vi "Create.vi"(8 "error in (no error)":errorcluster, 9 "multicast_ip":string="224.1.1.1", 10 "buffer":i32=10000, 11 "port":u16) -> (0 "error out":errorcluster, 3 "BME280 out":refnum<class "BME280.lvclass">)   [LabVIEW 2020, in "BME280.lvclass"]
uses:
  BME280.lvclass
  Weather.ctl
  BME280.lvclass/BME280.ctl
  <vilib>/Utility/tcp.llb/UDP Multicast Read-Only Open.vi
  __main.vi
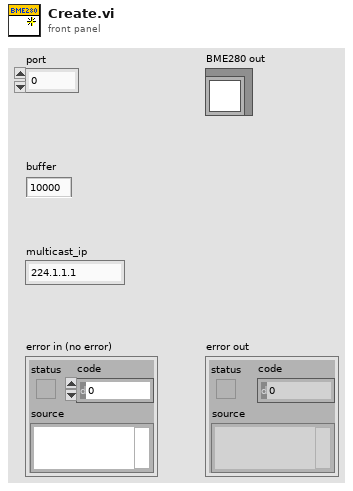
[diagram p1: front panel]
types:
  T1 = typedef "BME280.lvclass/Weather.ctl" = cluster{"temperature":dbl[], "humidity":dbl[], "pressure":dbl[]}
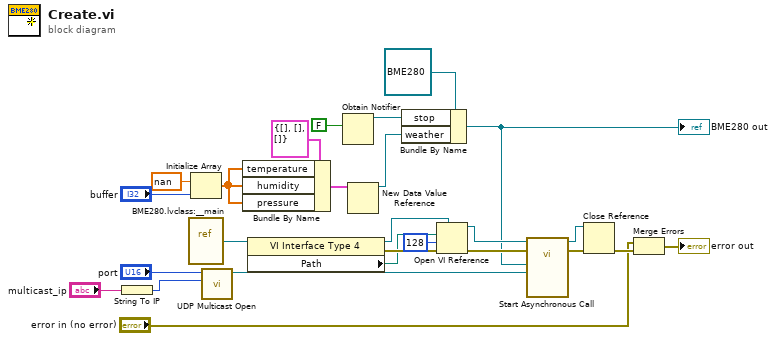
[diagram p0: block diagram]
diagram:
  n1 = String To IP(1:"multicast_ip") -> (0:w1:u32)
  n2 = vi-ref "BME280.lvclass:__main.vi"() -> (w17:refnum<vi>)
  n3 = Initialize Array(nan ("element"), "buffer") -> (w22:dbl[])
  n4 = call-poly <vilib>:"UDP Multicast Open.vi"("multicast addr"=w1, "port"="port") -> ("connection ID"=w2:refnum<k16>)  [unwired: 7 in, 2 out]
  n5 = Bundle By Name(cluster=T1 {"temperature"=[], "humidity"=[], "pressure"=[]} ("weather"), "temperature"=w22, "humidity"=w22, "pressure"=w22) -> (w21:T1)
  n6 = property class="VI Interface Type 4"(reference=w17) -> (reference out=w13:refnum<vi>, error out=w16:errorcluster, "Path"=w15:path)  [unwired: 1 in]
  n7 = Obtain Notifier(notification data type=FALSE) -> (notifier out=w18:refnum<notifier>)  [unwired: 3 in, 2 out]
  n8 = New Data Value Reference(data value=w21) -> (data value reference=w19:refnum<data-value>)  [unwired: 1 in, 1 out]
  n9 = Bundle By Name(cluster=refnum<class "BME280.lvclass"> refnum ("BME280.lvclass"), "stop"=w18, "weather"=w19) -> (w5:refnum<class "BME280.lvclass">)
  "BME280 out" <- w5
  n10 = Open VI Reference(type specifier VI Refnum (for type only)=w13, vi path=w15, options=128, error in (no error)=w16) -> (vi reference=w11:refnum<vi>, error out=w12:errorcluster)  [unwired: 2 in]
  n11 = call-by-ref "Start Asynchronous Call"(reference=w11, error in=w12, "udpCxcn"=w2, "BME280 in"=w5) -> (reference out=w9:refnum<vi>, error out=w10:errorcluster)  [unwired: 8 in, 2 out]
  n12 = Close Reference(reference=w9, error in (no error)=w10) -> (error out=w8:errorcluster)
  n13 = Merge Errors("error in (no error)", w8) -> (→"error out":errorcluster)
